vi "poly_data_queue_bool.vi"(7 "initialize":bool, 8 "error in":errorcluster caption="Error in (no error)", 9 "queue length (100)":i32=100, 10 "input data point":bool) -> (0 "error out":errorcluster, 1 "eliminated element":bool, 2 "queue":bool[](array[boolean]), 4 "current length":i32)   [LabVIEW 2015, in "_average_tools_polys.lvlib"]
uses:
  _average_tools_polys.lvlib
panel:
  in  "initial queue element (F)":bool
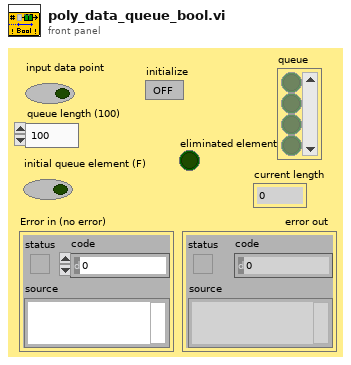
[diagram p1: front panel]
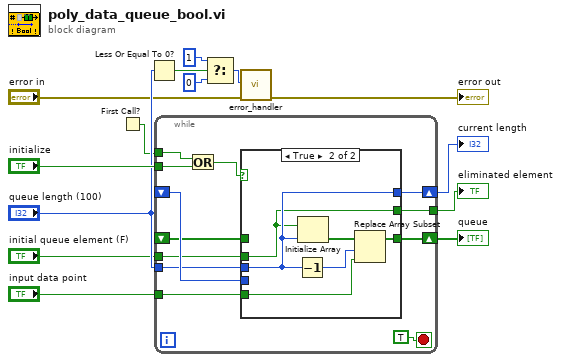
[diagram p0: block diagram]
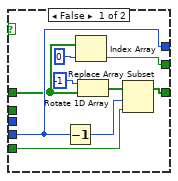
[diagram p2: hidden frame]
diagram:
  n1 = First Call?() -> (First Call?: T/F=w11:bool)
  n2 = Less Or Equal To 0?(x="queue length (100)") -> (x <= 0?=w10:bool)
  n3 = while {
    tunnel: w11 -> [w21]
    shift-left: _ -> [w24]
    shift-right: [w25] -> w14
    shift-left: _ -> [w23]
    shift-right: [w26] -> w2
    tunnel: "initialize" -> [w19]
    tunnel: "input data point" -> [w18]
    tunnel: "initial queue element (F)" -> [w17]
    tunnel: "queue length (100)" -> [w16]
    tunnel: [w15] -> w1
    stop <- TRUE stop-if-true
    n4 = Or(x=w21, y=w19) -> (x .or. y?=w20:bool)
    n5 = case shown="True" w20 {
      tunnel: [w32 w37] -> w26
      tunnel: [w33 w40] -> w25
      tunnel: w24 -> [w33 _]
      tunnel: w23 -> [w29 _]
      tunnel: w18 -> [w34 w38]
      tunnel: w17 -> [_ w36]
      tunnel: w16 -> [_ w40]
      tunnel: [w27 w36] -> w15
      frame False {
        n6 = Decrement(x=w33) -> (x-1=w31:i32)
        n7 = Index Array(array=w29, index=0 ("Index")) -> (element=w27:bool)
        n8 = Rotate 1D Array(1:w29, 2:i16 -1 ("n")) -> (0:w30:bool[])
        n9 = Replace Array Subset(array=w30, new element=w34, index=w31) -> (w32:bool[])
      }
      frame True {
        n10 = Decrement(x=w40) -> (x-1=w41:i32)
        n11 = Initialize Array(w36, w40) -> (w39:bool[])
        n12 = Replace Array Subset(array=w39, new element=w38, index=w41) -> (w37:bool[])
      }
    }
  }
  "current length" <- w14
  "queue" <- w2
  "eliminated element" <- w1
  n13 = Select(t=1, s=w10, f=0) -> (s? t:f=w7:i32)
  n14 = call "error_handler.vi"("error in (no error)"="error in", "code (0 = no error)"=w7) -> ("error out"=→"error out":errorcluster)  [unwired: 8 in, 1 out]
